vi "Monitor Heaters.vi"(8 "error in (no error)":errorcluster, 10 "Address (0)":i32, 11 "VISA resource name":refnum<visa-resource-name>) -> (0 "error out":errorcluster, 1 "heater output":dbl, 2 "num heaters":i32, 3 "VISA resource name out":refnum<visa-resource-name>, 5 "humidifying heater output":dbl)   [LabVIEW 2016, in "Environment Chamber.lvlib" / "Climatic Chamber.lvlib"]
doc: "<b>Heater output monitor</B>\n\nReturns the number of controllable heaters and their heater output values."
uses:
  Climatic Chamber.lvlib
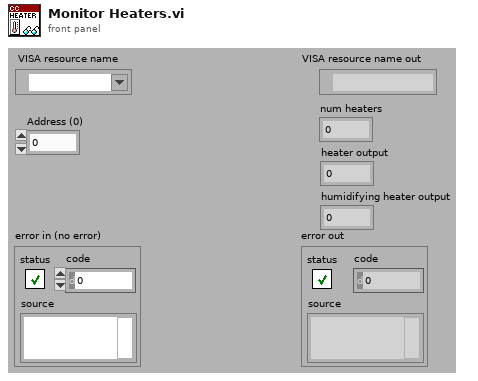
[diagram p1: front panel]
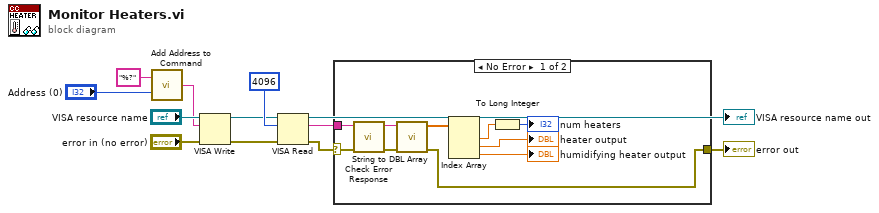
[diagram p0: block diagram]
diagram:
  n1 = call "Add Address to Command.vi"("Address (0)"="Address (0)", "Command"="%?") -> ("Command OUT"=w4:string)
  n2 = VISA Write(VISA resource name="VISA resource name", write buffer=w4, error in (no error)="error in (no error)") -> (VISA resource name out=w9:refnum<visa-resource-name>, error out=w8:errorcluster)  [unwired: 1 out]
  n3 = VISA Read(VISA resource name=w9, byte count=u32 4096, error in (no error)=w8) -> (VISA resource name out=→"VISA resource name out":refnum<visa-resource-name>, read buffer=w2:string, error out=w3:errorcluster)  [unwired: 1 out]
  n4 = case shown="No Error" w3 {
    selector: w3 -> [w16 w23]
    tunnel: w2 -> [w18 _]
    tunnel: [w14 w23] -> w1
    frame No Error {
      n5 = call "Check Error Response.vi"("error in (no error)"=w16, "read String"=w18) -> ("error out"=w15:errorcluster, "String out"=w17:string)  [unwired: 7 in, 1 out]
      n6 = call "String to DBL Array.vi"("error in (no error)"=w15, "String received"=w17) -> ("error out"=w14:errorcluster, "Array Data"=w22:dbl[])  [unwired: 8 in]
      n7 = Index Array(array=w22) -> (element #1=w21:dbl, element #2=→"heater output":dbl, element #3=→"humidifying heater output":dbl)  [unwired: 3 in]
      n8 = To Long Integer(number=w21) -> (32bit integer=→"num heaters":i32)
    }
    frame Error {
    }
  }
  "error out" <- w1
